vi "Write.vi"(8 "error in (no error)":errorcluster, 10 "Data":variant, 11 "DataShare in":refnum<class "DataShare.lvclass">) -> (0 "error out":errorcluster, 3 "DataShare out":refnum<class "DataShare.lvclass">)   [LabVIEW 2014, in "DataShare.lvclass"]
uses:
  DataShare.lvclass
  DataShare.lvclass/DataShare.ctl
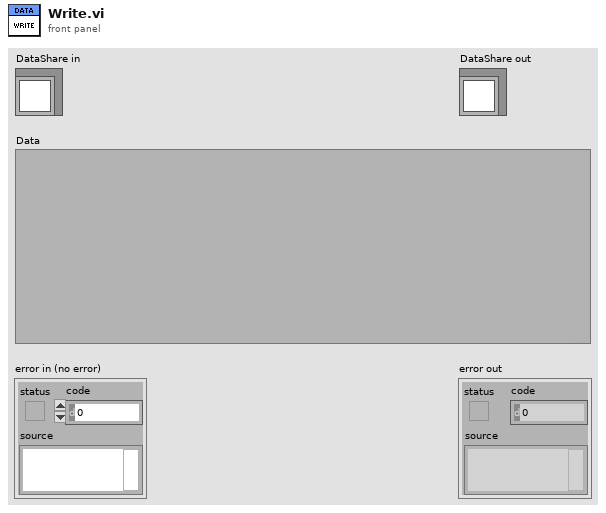
[diagram p1: front panel]
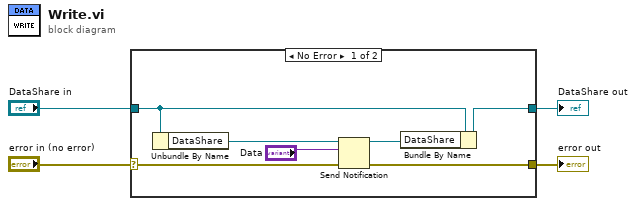
[diagram p0: block diagram]
diagram:
  n1 = case shown="No Error" "error in (no error)" {
    selector: "error in (no error)" -> [w10 w13]
    tunnel: [w9 w13] -> w3
    tunnel: [w6 w12] -> w1
    tunnel: "DataShare in" -> [w7 w12]
    frame No Error {
      n2 = Unbundle By Name(w7) -> ("DataShare"=w11:refnum<notifier>)
      n3 = Send Notification(notification="Data", notifier=w11, error in (no error)=w10) -> (notifier out=w8:refnum<notifier>, error out=w9:errorcluster)
      n4 = Bundle By Name(cluster=w7, "DataShare"=w8) -> (w6:refnum<class "DataShare.lvclass">)
    }
    frame Error {
    }
  }
  "error out" <- w3
  "DataShare out" <- w1
